vi "Generator.vi"(3 "Phase (0 °) (0 - 359.99)":dbl, 4 "Waveform (F) (F:Sine, T:Square)":bool, 5 "Frequency (125 Hz) (0.01 - 50e6)":dbl=125.0 format="%#_6p", 6 "Init (F)":bool, 7 "Voltage (2.5 V pp) (0.1 - 5)":dbl=2.5, 8 "error in (no error)":errorcluster) -> (0 "error out":errorcluster)   [LabVIEW 2019, in "ACSVcontrol-driver.lvlib"]
doc: "Set function generator. Init True will change the phase without a new initialisation, i.e. without switching to standby mode.\n\nInit true changes only frequency and phase, Amplitude input is irrelevant. If generator used, this VI must be run after PJVS.vi to reset phaselock signal."
uses:
  ACSVcontrol-driver.lvlib
  Private/Type definitions/Command.ctl
  Private/Type definitions/Status.ctl
  Private/Globals.vi
  <vilib>/Utility/error.llb/Error Cluster From Error Code.vi
  <vilib>/ErrorRing/Error Ring.xnode
panel:
  in  "number format string":string="%.6f"
  out "resulting string":string
  # ".7 is too much,\nworking maximum is .6"
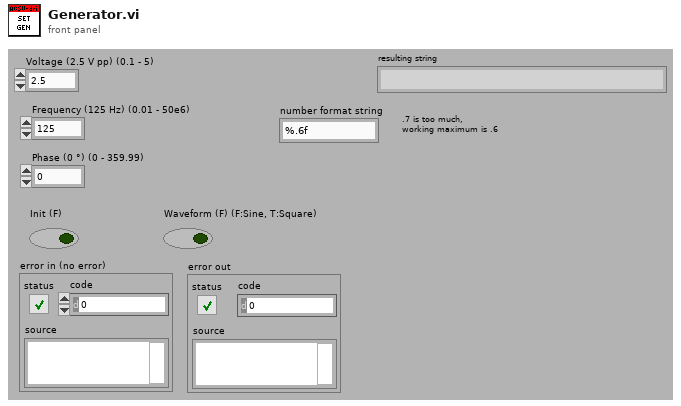
[diagram p1: front panel]
types:
  T1 = typedef "ACSVcontrol-driver.lvlib/Status.ctl" = enum16{"waiting", "processing", "error command", "Set_PJVS-Done", "Set_Mux-Done", "Set_Mux-Error", "Set_57XX-Done", "Set_57XX-Error", "Set_Gen-Done", "Set_Gen-Error", "Set_Synthesizer-Done", "Set_Synthesizer-Error", "Read_Nano-Done", "Read_Sampler-Done", "Read_Sampler-Error", "Read_Sensors-Done"}
  T2 = typedef "ACSVcontrol-driver.lvlib/Command.ctl" = enum16{"Set_PJVS", "Set_Mux", "Set_57XX", "Set_Gen", "Set_Synthesizer", "Read_Nulldetector", "Read_Sampler", "Read_Sensors"}
  T3 = typedef "ACSVcontrol-driver.lvlib/Timeouts.ctl" = cluster{"TCP Read & Write (ms)":i32, "Sensors readout":i32, "PJVS setup":i32, "Nullmeter readout":i32, "Multiplexer setup":i32, "57XX setup":i32, "Generator setup":i32, "Synthesizer setup":i32, "Sampler readout":i32}
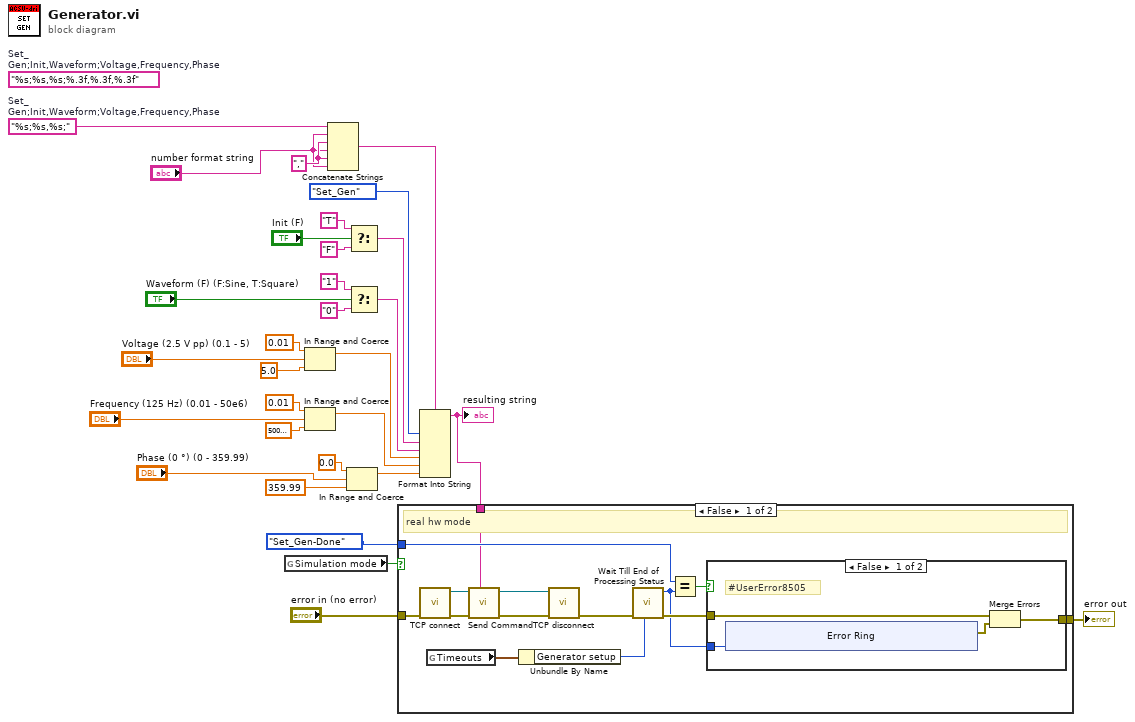
[diagram p0: block diagram]
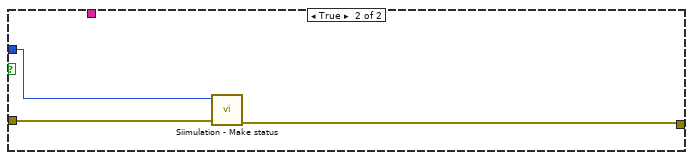
[diagram p3: hidden frame]
diagram:
  w6 = "%s;%s,%s;"  # Set_Gen;Init,Waveform;Voltage,Frequency,Phase
  w8 = "," ("string")
  (unwired) "%s;%s,%s;%.3f,%.3f,%.3f"  # Set_Gen;Init,Waveform;Voltage,Frequency,Phase
  n1 = global read "Globals.vi" "Simulation mode"() -> (w1:bool)
  n2 = In Range and Coerce(upper limit=0.01, x="Voltage (2.5 V pp) (0.1 - 5)", lower limit=5.0) -> (coerced(x)=w17:dbl)  [unwired: 1 out]
  n3 = In Range and Coerce(upper limit=0.01, x="Frequency (125 Hz) (0.01 - 50e6)", lower limit=50000000.0) -> (coerced(x)=w13:dbl)  [unwired: 1 out]
  n4 = Concatenate Strings(w6, "number format string", w8, "number format string", w8, "number format string") -> (w5:string)
  n5 = In Range and Coerce(upper limit=0.0, x="Phase (0 °) (0 - 359.99)", lower limit=359.99) -> (coerced(x)=w9:dbl)  [unwired: 1 out]
  n6 = Select(t="T" ("format string"), s="Init (F)", f="F" ("format string")) -> (s? t:f=w23:string)
  n7 = Select(t="1" ("format string"), s="Waveform (F) (F:Sine, T:Square)", f="0" ("format string")) -> (s? t:f=w22:string)
  n8 = Format Into String(format string=w5, Command."Set_Gen" ("Command"), w23, w22, w17, w13, w9) -> (resulting string=w2:string)  [unwired: 2 in, 1 out]
  "resulting string" <- w2
  n9 = case shown="False" w1 {
    tunnel: "error in (no error)" -> [w44 w59]
    tunnel: Status."Set_Gen-Done" ("x") -> [w38 w57]
    tunnel: [w37 w58] -> w3
    tunnel: w2 -> [w32 _]
    frame False {
      # "real hw mode"
      n10 = call "TCP connect.vi"("error in (no error)"=w44) -> ("error out"=w41:errorcluster, "connection ID"=w40:refnum<k5>)  [unwired: 9 in]
      n11 = global read "Globals.vi" "Timeouts"() -> (w31:T3)
      n12 = call "Send Command.vi"("Command"=w32, "error in (no error)"=w41, "connection ID"=w40) -> ("error out"=w42:errorcluster, "connection ID out"=w43:refnum<k5>)  [unwired: 7 in]
      n13 = Unbundle By Name(w31) -> ("Generator setup"=w33:i32)
      n14 = call "TCP disconnect.vi"("error in (no error)"=w42, "connection ID"=w43) -> ("error out"=w39:errorcluster)  [unwired: 9 in]
      n15 = call "Wait Till End of Processing Status.vi"("Loop Timeout (ms) (5000)"=w33, "error in (no error)"=w39) -> ("error out"=w36:errorcluster, "Last Status"=w34:T1)  [unwired: 8 in]
      n16 = Equal?(x=w38, y=w34) -> (x = y?=w35:bool)
      n17 = case shown="False" w35 {
        tunnel: w36 -> [w48 w56]
        tunnel: [w46 w56] -> w37
        tunnel: w34 -> [w45 _]
        frame False {
          # "#UserError8505"
          n18 = xnode "Error Ring"("parameter 0"=w45) -> ("error out"=w47:errorcluster)
          n19 = Merge Errors(w48, w47) -> (w46:errorcluster)
        }
        frame True {
        }
      }
    }
    frame True {
      n20 = call "Siimulation - Make status.vi"("error in (no error)"=w59, "Status"=w57) -> ("error out"=w58:errorcluster)  [unwired: 8 in, 1 out]
    }
  }
  "error out" <- w3
